vi "CAL_PRESSURE_TRANSDUCER.vi"(8 "error in (no error)":errorcluster, 11 "pressure_slope_IN":dbl=51.35 format="%.2f") -> (0 "error out":errorcluster, 3 "pressure_slope_OUT":dbl=51.35 format="%.2f")   [LabVIEW 2016]
uses:
  ad interface/Global_SIM_switch.vi
panel:
  out "ok":bool
  out "zero":bool
  out "Pressure":dbl format="%.2f"
  in  "ok":bool
  in  "zero":bool
  # "PRESSURE TRANSDUCER CALIBRATION"
  # "(step 1)"
  # "Fill graduated cylinder to 750 mL water.\nSubmerge Kpro effluent and start flow.\nStop flow at 800 mL of water (1 foot).\nAllow pressure to equilibrate and press zero."
  # "(step 2)"
  # "Hold Kpro effluent facing up and 5' above the floor.\nTurn Kpro flow on briefly to fill the Kpro line.\nTurn Kpro flow off again.\nPress OK when pressure has equilibrated"
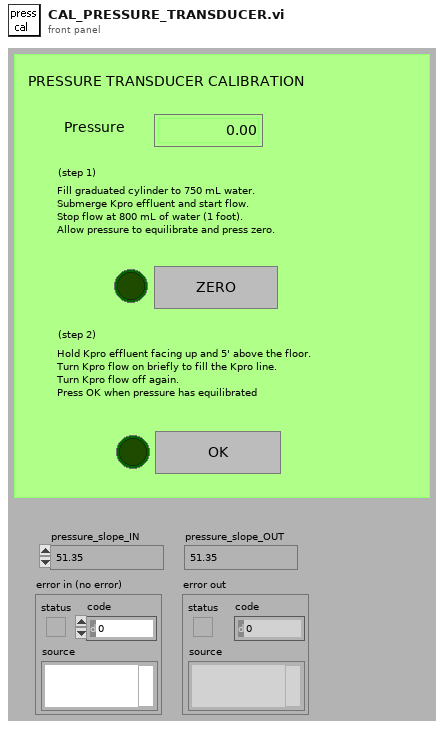
[diagram p1: front panel]
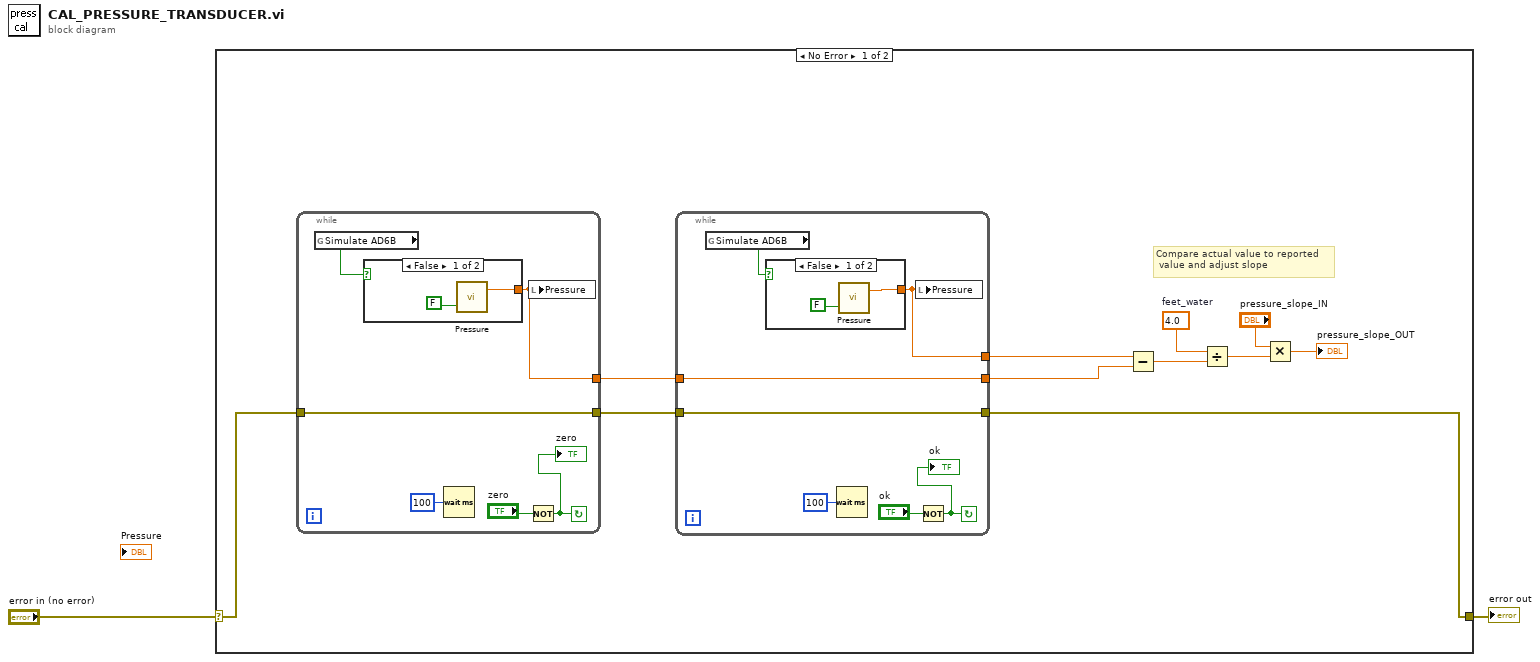
[diagram p0: block diagram]
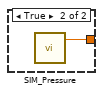
[diagram p2: hidden frame]
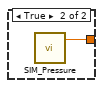
[diagram p3: hidden frame]
diagram:
  n1 = case shown="No Error" "error in (no error)" {
    selector: "error in (no error)" -> [w13 w33]
    tunnel: [w11 w33] -> w2
    frame No Error {
      w9 = 4.0  # feet_water
      # "Compare actual value to reported\n value and adjust slope"
      n2 = while {
        tunnel: [w16] -> w3
        tunnel: [w18] -> w12
        tunnel: w13 -> [w18]
        stop <- w14 continue-if-true
        n3 = global read "Global_SIM_switch.vi" "Simulate AD6B"() -> (w17:bool)
        n4 = case shown="False" w17 {
          tunnel: [w20 w22] -> w16
          frame False {
            n5 = call "Pressure.vi"("Zero Pressure\n(F = leave as is)"=FALSE ("Zero Pressure\n(F = leave as is)")) -> ("Pressure"=w20:dbl)  [unwired: 2 in]
          }
          frame True {
            n6 = call "SIM_Pressure.vi"() -> ("Pressure"=w22:dbl)  [unwired: 11 in]
          }
        }
        n7 = Wait (ms)(milliseconds to wait=u32 100) -> ()  [unwired: 1 out]
        n8 = Not(x="zero") -> (.not. x?=w14:bool)
        "zero" <- w14
        n9 = local write "Pressure"(w16) -> ()
      }
      n10 = while {
        tunnel: w3 -> [w26]
        tunnel: [w25] -> w6
        tunnel: [w26] -> w10
        tunnel: w12 -> [w27]
        tunnel: [w27] -> w11
        stop <- w23 continue-if-true
        n11 = global read "Global_SIM_switch.vi" "Simulate AD6B"() -> (w28:bool)
        n12 = case shown="False" w28 {
          tunnel: [w31 w32] -> w25
          frame False {
            n13 = call "Pressure.vi"("Zero Pressure\n(F = leave as is)"=FALSE ("Zero Pressure\n(F = leave as is)")) -> ("Pressure"=w31:dbl)  [unwired: 2 in]
          }
          frame True {
            n14 = call "SIM_Pressure.vi"() -> ("Pressure"=w32:dbl)  [unwired: 11 in]
          }
        }
        n15 = Wait (ms)(milliseconds to wait=u32 100) -> ()  [unwired: 1 out]
        n16 = local write "Pressure"(w25) -> ()
        n17 = Not(x="ok") -> (.not. x?=w23:bool)
        "ok" <- w23
      }
      n18 = Subtract(x=w6, y=w10) -> (x-y=w5:dbl)
      n19 = Divide(x=w9, y=w5) -> (x/y=w4:dbl)
      n20 = Multiply(x="pressure_slope_IN", y=w4) -> (x*y=→"pressure_slope_OUT":dbl)
    }
    frame Error {
    }
  }
  "error out" <- w2
